vi "Collector Controller Held Logic.vi"(10 "Button B":bool, 11 "Button A":bool) -> (3 "State out":T1=enum."Collector Motor Stop")   [LabVIEW 2016]
uses:
  Sprocket/src/Action/Action Name.ctl
  Sprocket/src/Refname/Actuators.ctl
  Sprocket/lib/Sprocket.lvlib
panel:
  in  "OverCurrent":dbl=30.0
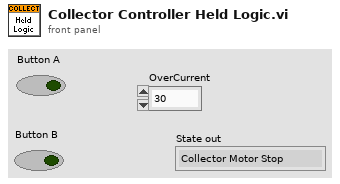
[diagram p1: front panel]
types:
  T1 = typedef "Sprocket.lvlib/Action Name.ctl" = enum16{"No Action", "Drive Train Both", "Drive Train Rotate", "Drive Train Throttle", "Collector Motor Roll", "Collector Motor Eject", "Collector Motor Collect", "Collector Motor Stop", "Collector Extend", "Collector Retract", "Shifter High", "Shifter Low", "Collector Motor Stall", "Wedge Roll"}
  T2 = typedef "Sprocket.lvlib/Actuators.ctl" = enum16{"Drive Motor 1 (R)", "Drive Motor 2 (R)", "Drive Motor 3 (R)", "Drive Motor 4 (L)", "Drive Motor 5 (L)", "Drive Motor 6 (L)", "Collector Motor", "Collector Solenoid", "Compressor", "SonicShifter", "Gyro", "UltraSonic Front Left", "UltraSonic Back Left", "Wedge Motor", "Wedge LS"}
  T3 = typedef "WPI_MotorControlDeviceRef.ctl" = cluster{"DeviceStatus":errorcluster, "Type":T4, "PWM":cluster{"PWM Channel":T5, "DeadBand":T6}, "CAN":cluster{"Device Number":u8, "SetOutput VI Ref":variant, "GetOutput VI Ref":variant, "Enable VI Ref":variant, "Disable VI Ref":variant, "Data":variant}, "Invert":bool}
  T4 = typedef "WPI_MotorControlType.ctl" = enum16{"PWM", "CAN"}
  T5 = typedef "FPGA_DIOPWMChannel.ctl" = enum8{"PWM 0", "PWM 1", "PWM 2", "PWM 3", "PWM 4", "PWM 5", "PWM 6", "PWM 7", "PWM 8", "PWM 9", "PWM MXP 0", "PWM MXP 1", "PWM MXP 2", "PWM MXP 3", "PWM MXP 4", "PWM MXP 5", "PWM MXP 6", "PWM MXP 7", "PWM MXP 8", "PWM MXP 9", "Invalid"}
  T6 = typedef "WPI_PWMDeadband.ctl" = cluster{"Name":string, "maxPositivePwm":i32, "minPositivePwm":i32, "centerPwm":i32, "maxNegativePwm":i32, "minNegativePwm":i32, "angularRange":u16}
  T7 = typedef "WPI_CANTalonSRX_GlobalStatus.ctl" = cluster{"Applied Throttle":dbl, "Module Enabled":bool, "CAN Error":errorcluster, "Closed Loop Error":dbl, "Forward Limit Switch Closed":bool, "Reverse Limit Switch Closed":bool, "Sensor Position":dbl, "Sensor Velocity":dbl, "Current":dbl, "Sticky Fault - Over Temp":bool, "Sticky Fault - Under Voltage":bool, "Sticky Fault - Forward Limit":bool, "Sticky Fault - Reverse Limit":bool, "Sticky Fault - Forward Soft Limit":bool, "Sticky Fault - Reverse Soft Limit":bool, "Brake is Enabled":bool, "Encoder Position":dbl, "Encoder Velocity":dbl, "Encoder Index Count":dbl, "Encoder A Pin State":bool, "Encoder B Pin State":bool, "Encoder Index Pin State":bool, "Analog In":dbl, "Analog In Velocity":dbl, "Temperature (C)":dbl, "Battery Voltage":dbl, "Control 5 Is Supported":bool, "Current Profile Slot Select":dbl, "Pos Div 8":bool, "Vel Div 4":bool, "Pulse Width Position":i32, "Pulse Width Velocity":i32, "Pulse Width Rise To Rise (us)":i32, "Pulse Width Rise To Fall (us)":i32, "Mot Prof Active Is Under Run":bool, "Mot Prof Active Has Under Run":bool, "Mot Prof Active Is Last":bool, "Mot Prof Active Velocity Only":bool, "Mot Prof Active Is Valid":bool, "Mot Prof Buffer Is Full":bool, "Mot Prof Active Profile Slot Select":i32, "Mot Prof NextID":i32, "Mot Prof Count":i32, "Mot Prof Active Velocity":dbl, "Mot Prof Active Position":dbl, "Mot Prof Output Enable":i32}
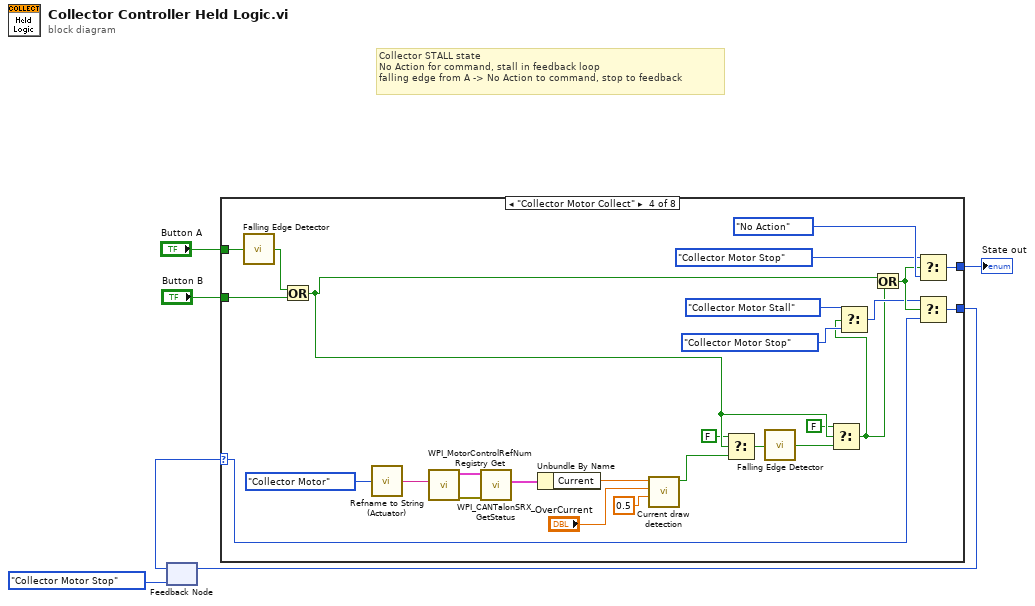
[diagram p0: block diagram]
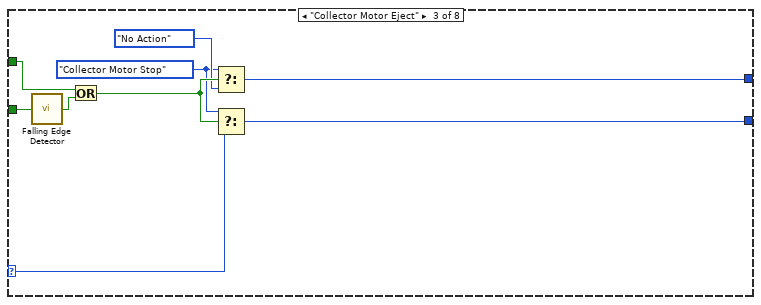
[diagram p4: hidden frame]
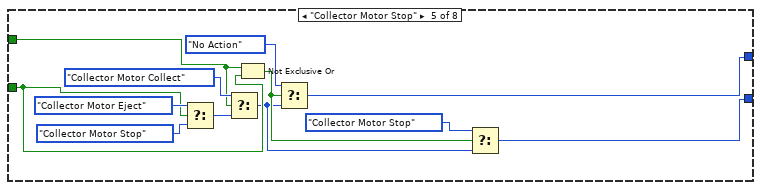
[diagram p5: hidden frame]
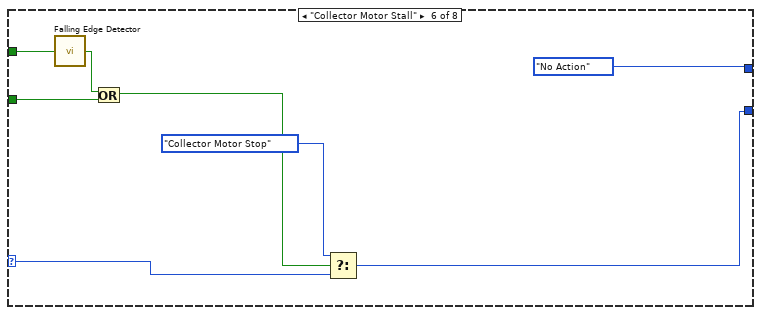
[diagram p6: hidden frame]
diagram:
  # "Collector STALL state\nNo Action for command, stall in feedback loop\nfalling edge from A -> No Action to command, stop to feedback"
  n1 = feedback #1(Action_Name."Collector Motor Stop" ("Name")) -> (w1:T1)
  n2 = case shown="\"Collector Motor Collect\"" w1 {
    selector: w1 -> [w7 w8 w15 w42 _ w60 w65 w66]
    tunnel: "Button A" -> [_ _ w10 w44 w51 w63 _ _]
    tunnel: "Button B" -> [_ _ w16 w37 w52 w62 _ _]
    tunnel: [w7 w8 w14 w43 w45 w59 w65 w66] -> w3
    tunnel: [w7 w8 w13 w41 w49 Action_Name."No Action" ("Name") w65 w66] -> w4
    frame "No Action", Default {
    }
    frame "Collector Motor Roll" {
    }
    frame "Collector Motor Eject" {
      w11 = Action_Name."Collector Motor Stop" ("Name")
      n3 = call "Falling Edge Detector.vi"("Input"=w16) -> ("Falling edge?"=w9:bool)
      n4 = Or(x=w10, y=w9) -> (x .or. y?=w17:bool)
      n5 = Select(t=w11, s=w17, f=Action_Name."No Action" ("Name")) -> (s? t:f=w13:T1)
      n6 = Select(t=w11, s=w17, f=w15) -> (s? t:f=w14:T1)
    }
    frame "Collector Motor Collect" {
      n7 = call "Falling Edge Detector.vi"("Input"=w44) -> ("Falling edge?"=w38:bool)
      n8 = Or(x=w38, y=w37) -> (x .or. y?=w32:bool)
      n9 = call "Refname to String (Actuator).vi"("Actuator Refname"=Actuators."Collector Motor") -> ("Refnum Name"=w28:string)
      n10 = call <vilib>:"WPI_MotorControlRefNum Registry Get.vi"("refnum name"=w28) -> ("error out"=w26:errorcluster, "MotorControlDevRef"=w27:T3)  [unwired: 9 in]
      n11 = call <vilib>:"WPI_CANTalonSRX_GetStatus.vi"("error in (no error)"=w26, "CAN Talon SRX Ref"=w27) -> ("Talon SRX Status"=w30:T7)  [unwired: 7 in, 2 out]
      n12 = Unbundle By Name(w30) -> ("Current"=w18:dbl)
      n13 = call "Current draw detection.vi"("Time to Free spin (s)"=0.5, "OverCurrent"="OverCurrent", "Current"=w18) -> ("Normal?"=w21:bool)  [unwired: 8 in]
      n14 = Select(t=FALSE, s=w32, f=w21) -> (s? t:f=w25:bool)
      n15 = call "Falling Edge Detector.vi"("Input"=w25) -> ("Falling edge?"=w24:bool)
      n16 = Select(t=FALSE, s=w32, f=w24) -> (s? t:f=w31:bool)
      n17 = Select(t=Action_Name."Collector Motor Stall" ("Name"), s=w31, f=Action_Name."Collector Motor Stop" ("Name")) -> (s? t:f=w34:T1)
      n18 = Or(x=w32, y=w31) -> (x .or. y?=w36:bool)
      n19 = Select(t=Action_Name."Collector Motor Stop" ("Name"), s=w36, f=Action_Name."No Action" ("Name")) -> (s? t:f=w41:T1)
      n20 = Select(t=w34, s=w36, f=w42) -> (s? t:f=w43:T1)
    }
    frame "Collector Motor Stop" {
      n21 = Select(t=Action_Name."Collector Motor Eject" ("Name"), s=w52, f=Action_Name."Collector Motor Stop" ("Name")) -> (s? t:f=w54:T1)
      n22 = Select(t=Action_Name."Collector Motor Collect" ("Name"), s=w51, f=w54) -> (s? t:f=w46:T1)
      n23 = Not Exclusive Or(1:w52, 2:w51) -> (0:w48:bool)
      n24 = Select(t=Action_Name."No Action" ("Name"), s=w48, f=w46) -> (s? t:f=w49:T1)
      n25 = Select(t=Action_Name."Collector Motor Stop" ("Name"), s=w48, f=w46) -> (s? t:f=w45:T1)
    }
    frame "Collector Motor Stall" {
      n26 = call "Falling Edge Detector.vi"("Input"=w63) -> ("Falling edge?"=w64:bool)
      n27 = Or(x=w64, y=w62) -> (x .or. y?=w61:bool)
      n28 = Select(t=Action_Name."Collector Motor Stop" ("Name"), s=w61, f=w60) -> (s? t:f=w59:T1)
    }
    frame "Collector Extend" {
    }
    frame "Collector Retract" {
    }
  }
  "State out" <- w4
  n29 = feedback-in #1(w3) -> ()
